vi "ReadConfig.vi"(8 "error in (no error)":errorcluster, 11 "GRMActor in":refnum<class "QPDController.lvclass">) -> (0 "error out":errorcluster, 3 "GRMActor out":refnum<class "QPDController.lvclass">)   [LabVIEW 2020, in "QPDController.lvlib" / "QPDController.lvclass"]
uses:
  QPDController.lvclass
  QPDController.lvclass/QPDController.ctl
  Model/Hardware Abstraction Layer/Component/GenericActor/GenericActor/GenericController.lvclass
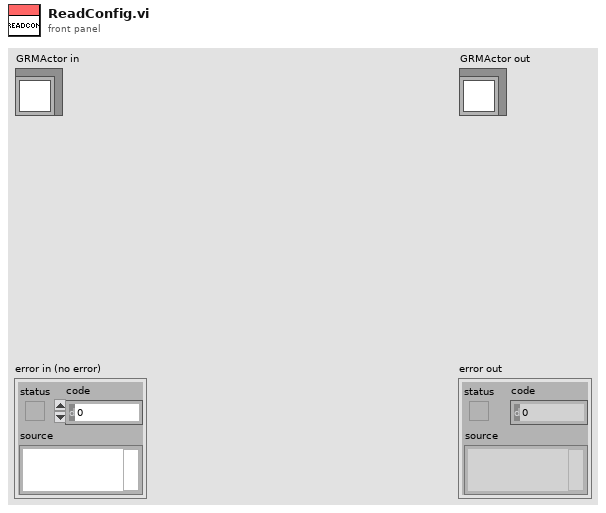
[diagram p1: front panel]
types:
  T1 = typedef "NI_LVConfig.lvlib/Config Data RefNum.ctl" = refnum<k1>
  T2 = cluster{"Values[0]":dbl, "Values[1]":dbl, "Values[2]":dbl, "Values[3]":dbl}
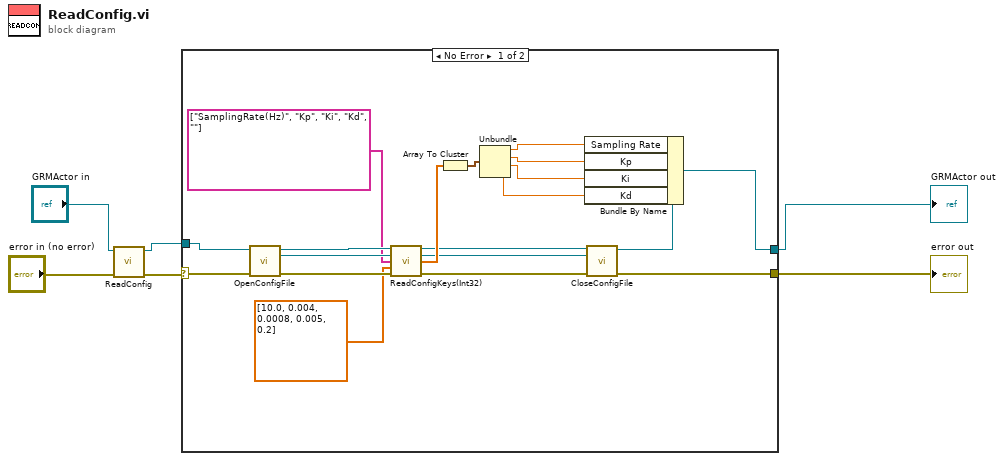
[diagram p0: block diagram]
diagram:
  n1 = call-parent "ReadConfig.vi"("error in (no error)"="error in (no error)", "GRMActor in"="GRMActor in") -> ("error out"=w4:errorcluster, "GRMActor out"=w3:refnum<class "QPDController.lvclass">)  [unwired: 8 in]
  n2 = case shown="No Error" w4 {
    selector: w4 -> [w25 w26]
    tunnel: [w17 w26] -> w1
    tunnel: [w20 w27] -> w2
    tunnel: w3 -> [w24 w27]
    frame No Error {
      n3 = call-dynamic "OpenConfigFile.vi"("error in (no error)"=w25, "GRMActor in"=w24) -> ("error out"=w23:errorcluster, "refnum"=w18:T1, "GRMActor out"=w21:refnum<class "QPDController.lvclass">)  [unwired: 7 in]
      n4 = call-dynamic "ReadConfigKeys(Int32).vi"("GRMActor in"=w21, "Config Refnum"=w18, "Keys"=string[] ["SamplingRate(Hz)", "Kp", "Ki", "Kd", ""] ("Values"), "Default"=dbl[] [10.0, 0.004, 0.0008, 0.005, 0.2], "error in (no error)"=w23) -> ("GRMActor out"=w13:refnum<class "QPDController.lvclass">, "Config Refnum dup"=w12:T1, "Values"=w15:dbl[], "error out"=w22:errorcluster)  [unwired: 7 in]
      n5 = Array To Cluster(array=w15) -> (cluster=w19:T2)
      n6 = Unbundle(w19) -> ("Values[0]"=w10:dbl, "Values[1]"=w9:dbl, "Values[2]"=w8:dbl, "Values[3]"=w7:dbl)
      n7 = call-dynamic "CloseConfigFile.vi"("error in (no error)"=w22, "refnum"=w12, "GRMActor in"=w13) -> ("error out"=w17:errorcluster, "GRMActor out"=w16:refnum<class "QPDController.lvclass">)  [unwired: 7 in]
      n8 = Bundle By Name(cluster=w16, "Sampling Rate"=w10, "Kp"=w9, "Ki"=w8, "Kd"=w7) -> (w20:refnum<class "QPDController.lvclass">)
    }
    frame Error {
    }
  }
  "error out" <- w1
  "GRMActor out" <- w2
